vi "Add Message Section.vi"(8 "error in":errorcluster, 10 "message section name":string, 11 "bus controller":T1 format="%.0x") -> (0 "error out":errorcluster, 2 "message section":T1 format="%.0x", 3 "bus controller out":T1 format="%.0x")   [LabVIEW 2020, in "AIM MIL-STD-1553 Scripting.lvlib"]
doc: "Adds a Message Section to the specified <b>bus controller</b> using the name in <b>message name</b> and returns a reference to the added <b>message section</b>."
uses:
  AIM MIL-STD-1553 Scripting.lvlib
  <vilib>/NI VeriStand/Custom Device API/Custom Device API.lvlib
  Constants.vi
  <vilib>/NI VeriStand/Custom Device API/Custom Device Item Ref.ctl
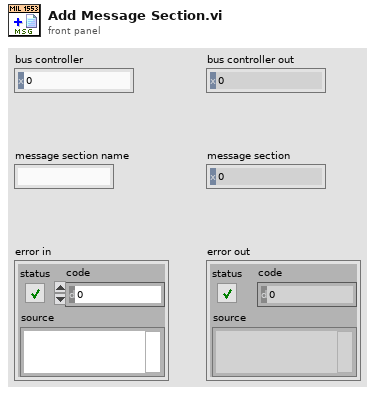
[diagram p1: front panel]
types:
  T1 = typedef "Custom Device API.lvlib/Custom Device Item Ref.ctl" = u64
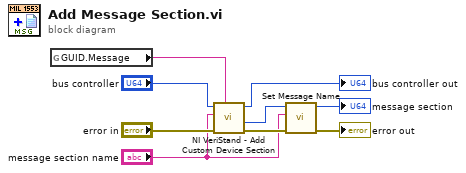
[diagram p0: block diagram]
diagram:
  n1 = global read "Constants.vi" "GUID.Message"() -> (w9:string)
  n2 = call <vilib>:"NI VeriStand - Add Custom Device Section.vi"("GUID (Default Section)"=w9, "error in (no error)"="error in", "Section Name"="message section name", "Parent Ref in"="bus controller") -> ("error out"=w5:errorcluster, "Section Ptr"=w6:T1, "Parent Ref out"=→"bus controller out":T1)  [unwired: 4 in, 1 out]
  n3 = call "Set Message Name.vi"("error in"=w5, "name"="message section name", "message or subaddress"=w6) -> ("error out"=→"error out":errorcluster, "message or subaddress out"=→"message section":T1)  [unwired: 7 in]
